vi "XNET Read (Frame FlexRay).vi"(0 "session in":refnum<k21>, 7 "number to read (-1)":i32=-1, 9 "timeout (0)":dbl format="%.2g", 11 "error in (no error)":errorcluster) -> (4 "session out":refnum<k21>, 6 "data":T1[](array[typedef]) {"payload" format="%x"; "timestamp" format="%<%.7X\n%x>T"; "type" items=["FlexRay Data"=32, "FlexRay Null"=33, "FlexRay Symbol"=34, "Log Trigger"=225, "Start Trigger"=226]; "cycle count" max=63 step=1}, 14 "unused payloads":cluster{"payload":u8[]}[](array[cluster]), 15 "error out":errorcluster)   [LabVIEW 2018]
doc: "Reads data from a session as an array of FlexRay frames. The session must use a FlexRay interface and a mode of Frame Input Stream, Frame Input Queued, or Frame Input Single-Point."
uses:
  XNET Frame FlexRay.ctl
  XNET Frame Type FlexRay.ctl
  nixlvapi.dll
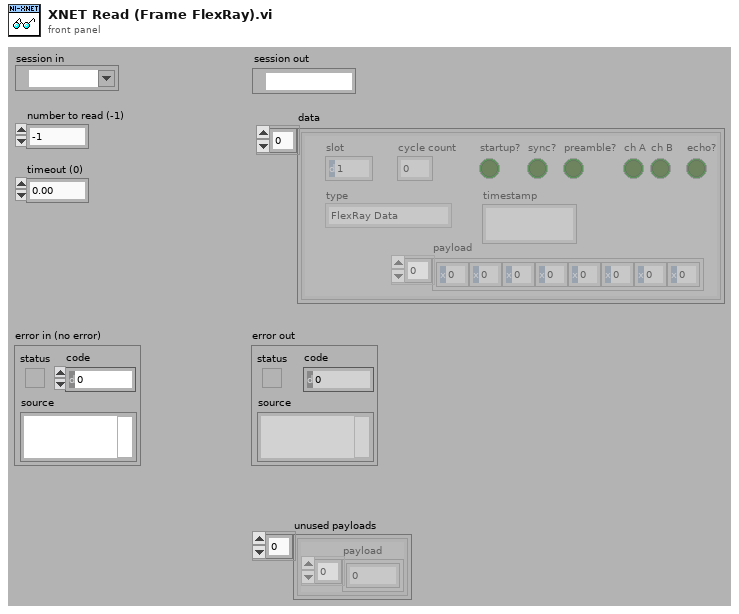
[diagram p1: front panel]
types:
  T1 = typedef "XNET Frame FlexRay.ctl" = cluster{"timestamp":timestamp, "payload":u8[], "slot":u16, "type":T2, "cycle count":u8, "startup?":bool, "sync?":bool, "preamble?":bool, "ch A":bool, "ch B":bool, "echo?":bool}
  T2 = typedef "XNET Frame Type FlexRay.ctl" = u8
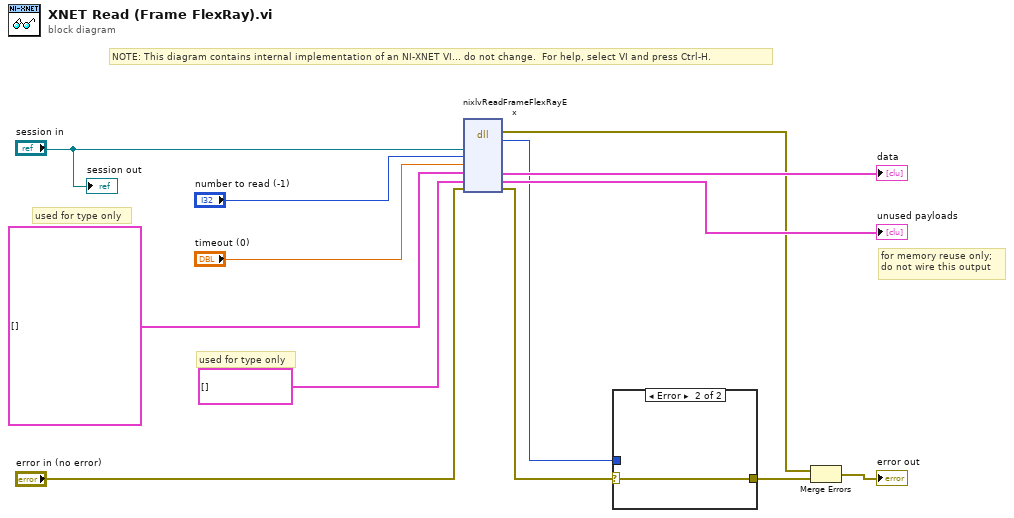
[diagram p0: block diagram]
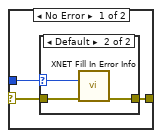
[diagram p2: hidden frame]
diagram:
  # "for memory reuse only;\ndo not wire this output"
  # "used for type only"
  # "used for type only"
  # "NOTE: This diagram contains internal implementation of an NI-XNET VI... do not change.  For help, select VI and press Ctrl-H."
  n1 = dll-call lib="nixlvapi.*" fn="nixlvReadFrameFlexRayEx" label="Call Library"("sessionRef"="session in", "numberToRead"="number to read (-1)", "timeout"="timeout (0)", "lvData"=T1[] [] ("data"), "unusedPayloads"=cluster{"payload":u8[]}[] [] ("payload array"), "errorInOut"="error in (no error)") -> (error out=w1:errorcluster, "return type"=w4:i32, "lvData"=→"data":T1[], "unusedPayloads"=→"unused payloads":cluster{"payload":u8[]}[], "errorInOut"=w3:errorcluster)  [unwired: 5 in, 2 out]
  n2 = case shown="Error" w3 {
    selector: w3 -> [w14 w21]
    tunnel: [w16 w21] -> w13
    tunnel: w4 -> [w15 _]
    frame No Error {
      n3 = case shown="Default" w15 {
        selector: w15 -> [_ w18]
        tunnel: w14 -> [w17 w19]
        tunnel: [w17 w20] -> w16
        frame 0 {
        }
        frame Default {
          n4 = call "XNET Fill In Error Info.vi"("status code"=w18, "error in"=w19) -> ("error out"=w20:errorcluster)  [unwired: 13 out]
        }
      }
    }
    frame Error {
    }
  }
  n5 = Merge Errors(w1, w13) -> (→"error out":errorcluster)
  "session out" <- "session in"
